vi "Set Method End Time.vi"(9 "Method Start Time":timestamp, 10 "Test Method Name":string, 11 "Test Case Result In":refnum<class "Test Case Result.lvclass">) -> (3 "Test Case Result Out":refnum<class "Test Case Result.lvclass">)   [LabVIEW 2020, in "Test Case Result.lvclass"]
uses:
  Test Case Result.lvclass
  Test Case Result.lvclass/Test Case Result.ctl
  Method Result/Method Result.lvclass/Method Result.ctl
  Method Result/Method Result.lvclass
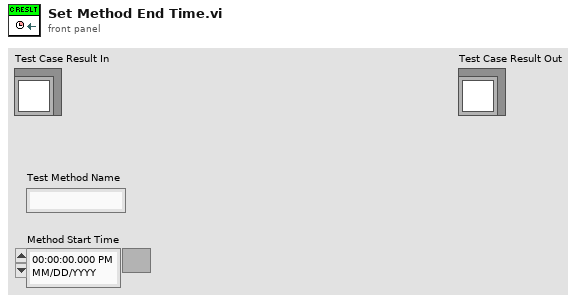
[diagram p1: front panel]
types:
  T1 = map{string, refnum<class "Method Result.lvclass">}
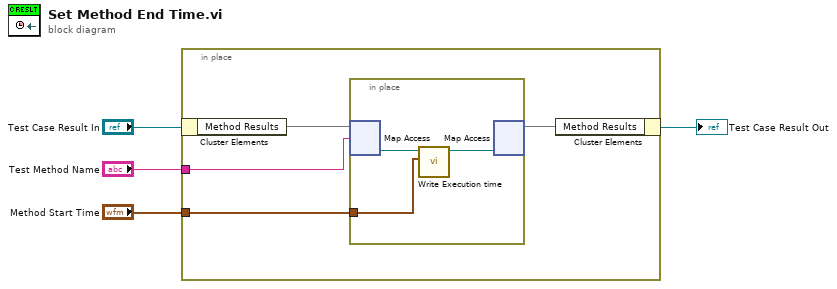
[diagram p0: block diagram]
diagram:
  n1 = in-place {
    in-place-border: "Test Method Name" -> [w7]
    in-place-border: "Method Start Time" -> [w6]
    n2 = in-place-cluster #1("Test Case Result In") -> ("Method Results"=w8:T1)
    n3 = in-place {
      in-place-border: w6 -> [w11]
      n4 = in-place-map #2(w8, w7) -> (w10:refnum<class "Method Result.lvclass">)  [unwired: 1 in, 1 out]
      n5 = call "Write Execution time.vi"("Method Start Time"=w11, "Method Result In"=w10) -> ("Method Result Out"=w9:refnum<class "Method Result.lvclass">)  [unwired: 9 in]
      n6 = in-place-map #2(w9) -> (w5:T1)  [unwired: 1 in, 2 out]
    }
    n7 = in-place-cluster #1("Method Results"=w5) -> (→"Test Case Result Out":refnum<class "Test Case Result.lvclass">)
  }
